vi "setScriptEvent.vi"(8 "error in (no error)":errorcluster, 10 "ScriptEvent.lvclass":refnum<class "ScriptEvent.lvclass">, 11 "ActionPanel.lvclass in":refnum<class "ActionPanel.lvclass">) -> (0 "error out":errorcluster, 3 "ActionPanel.lvclass out":refnum<class "ActionPanel.lvclass">)   [LabVIEW 2009, in "Views.lvlib" / "ScriptEditor.lvlib" / "ActionPanel.lvclass"]
uses:
  ActionPanel.lvclass
  Tools/Scripting/ScriptingEvent/ScriptEvent.lvclass
  ActionPanel.lvclass/ActionPanel.ctl
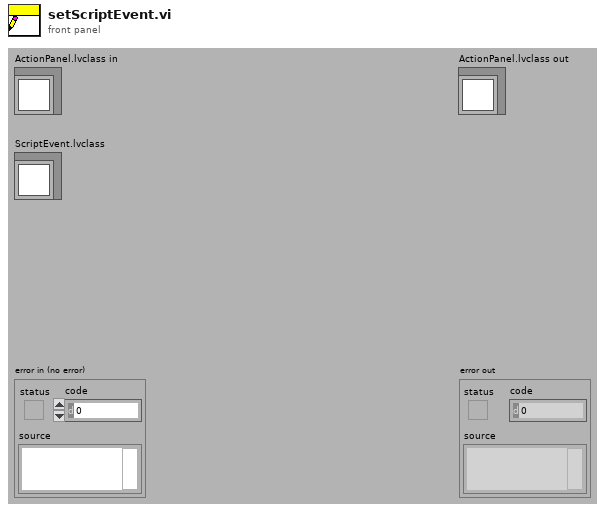
[diagram p1: front panel]
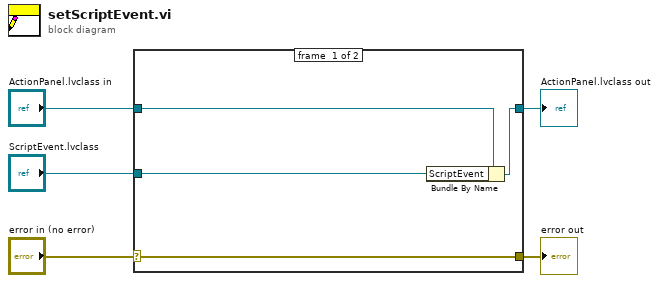
[diagram p0: block diagram]
diagram:
  n1 = case shown="No Error" "error in (no error)" {
    selector: "error in (no error)" -> [w9 w10]
    tunnel: [w9 w10] -> w4
    tunnel: [w7 w11] -> w2
    tunnel: "ActionPanel.lvclass in" -> [w8 w11]
    tunnel: "ScriptEvent.lvclass" -> [w6 _]
    frame #0 {
      n2 = Bundle By Name(cluster=w8, "ScriptEvent"=w6) -> (w7:refnum<class "ActionPanel.lvclass">)
    }
    frame #1 {
    }
  }
  "error out" <- w4
  "ActionPanel.lvclass out" <- w2
